vi "distance formula FINAL 30.vi"(8 "Y Seconds":dbl, 10 "inSpeed":dbl format="%#_13g", 11 "X Seconds":dbl) -> (0 "Seconds":dbl, 2 "outSpeed":dbl format="%#_13g", 3 "Hypotenuse Degrees":dbl)   [LabVIEW 2014]
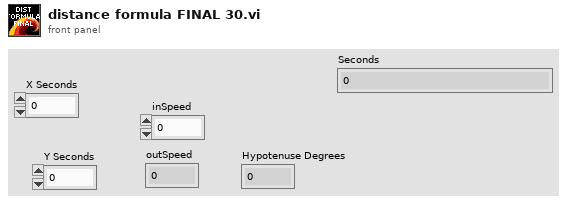
[diagram p1: front panel]
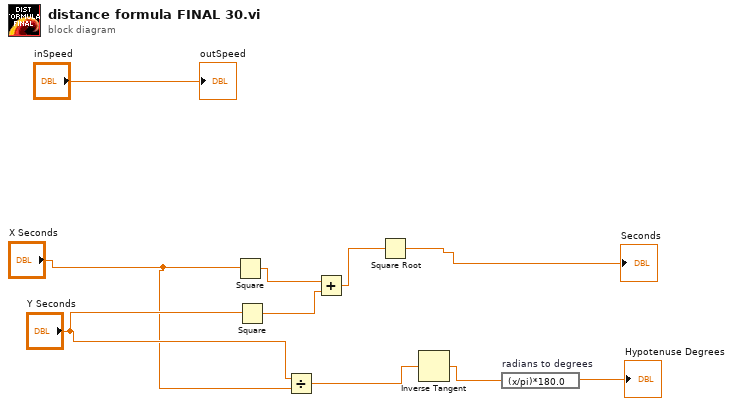
[diagram p0: block diagram]
diagram:
  n1 = Square(x="X Seconds") -> (x^2=w9:dbl)
  n2 = Square(x="Y Seconds") -> (x^2=w10:dbl)
  n3 = Divide(x="Y Seconds", y="X Seconds") -> (x/y=w4:dbl)
  n4 = Add(x=w9, y=w10) -> (x+y=w8:dbl)
  n5 = Square Root(x=w8) -> (sqrt(x)=→"Seconds":dbl)
  n6 = Inverse Tangent(1:w4) -> (0:w3:dbl)
  n7 = expression code="(x/pi)*180.0" "radians to degrees"(w3) -> (→"Hypotenuse Degrees":dbl)
  "outSpeed" <- "inSpeed"
